vi "MongoDB.JSONtoQueryDoc.vi"(8 "error in (no error)":errorcluster, 11 "JSON Query String":string) -> (0 "error out":errorcluster, 3 ".NET Refnum out":refnum<k24>)   [LabVIEW 2014]
uses:
  C:/Users/Richard/Documents/GitHub/mongo-labview-driver/CSharp/bin/MongoDB.Driver.Legacy.dll
  CSharp/bin/MongoDB.Driver.Legacy.dll
  C:/Users/Richard/Documents/GitHub/mongo-labview-driver/CSharp/bin/MongoDB.Bson.dll
  CSharp/bin/MongoDB.Bson.dll
panel:
  out "error out 2":errorcluster
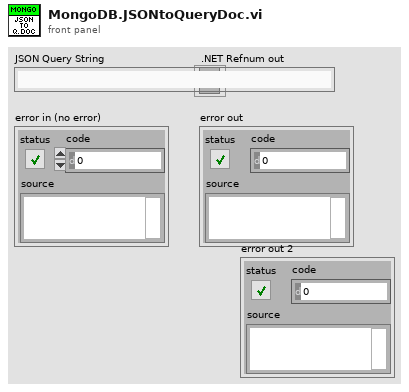
[diagram p1: front panel]
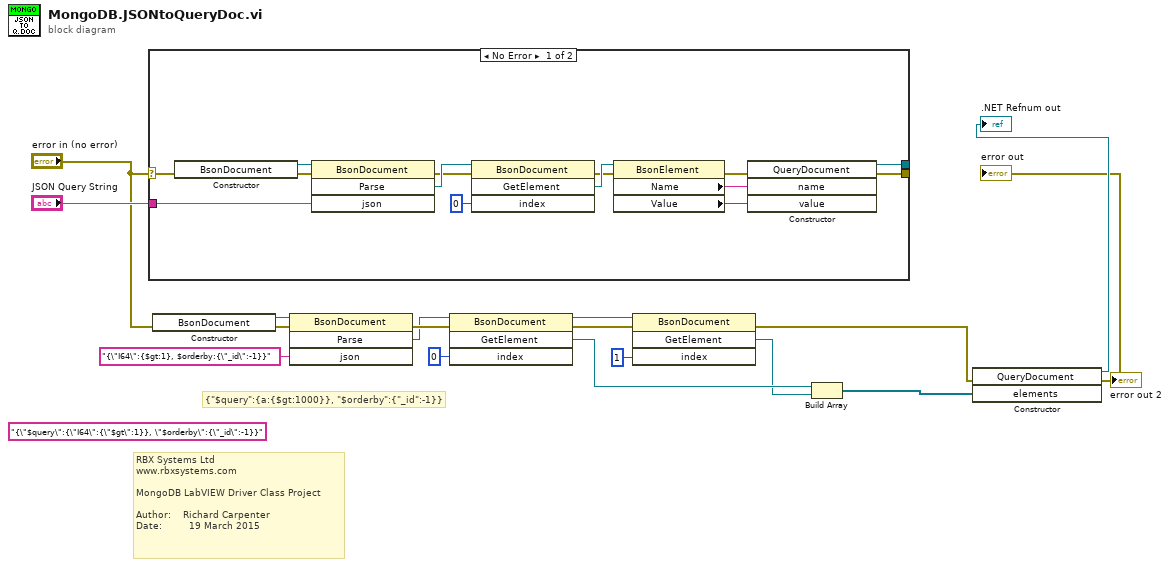
[diagram p0: block diagram]
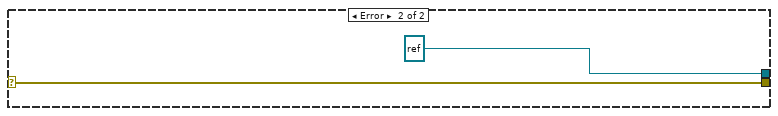
[diagram p2: hidden frame]
diagram:
  (unwired) "{\"$query\":{\"I64\":{\"$gt\":1}}, \"$orderby\":{\"_id\":-1}}" ("json")
  # "{\"$query\":{a:{$gt:1000}}, \"$orderby\":{\"_id\":-1}}"
  # "RBX Systems Ltd\nwww.rbxsystems.com\n\nMongoDB LabVIEW Driver Class Project\n\nAuthor:    Richard Carpenter\nDate:         19 March 2015"
  n1 = case shown="No Error" "error in (no error)" {
    selector: "error in (no error)" -> [w18 w33]
    tunnel: [w31 w33] -> _
    tunnel: [w30 refnum<k24> refnum ("new reference")] -> _
    tunnel: "JSON Query String" -> [w29 _]
    frame No Error {
      n2 = constructor class="BsonDocument"(error in=w18) -> (reference out=w20:refnum<k24>, error out=w19:errorcluster)  [unwired: 2 in, 1 out]
      n3 = invoke class="BsonDocument" method="Parse"(reference=w20, error in=w19, "json"=w29) -> (error out=w21:errorcluster, "Parse"=w28:refnum<k24>)  [unwired: 1 in, 2 out]
      n4 = invoke class="BsonDocument" method="GetElement"(reference=w28, error in=w21, "index"=0) -> (error out=w22:errorcluster, "GetElement"=w27:refnum<k24>)  [unwired: 1 in, 2 out]
      n5 = property class="BsonElement"(reference=w27, error in=w22) -> (error out=w23:errorcluster, "Name"=w25:string, "Value"=w26:refnum<k24>)  [unwired: 1 out]
      n6 = constructor class="QueryDocument"(error in=w23, "name"=w25, "value"=w26) -> (reference out=w30:refnum<k24>, error out=w31:errorcluster)  [unwired: 2 in, 3 out]
    }
    frame Error {
    }
  }
  n7 = constructor class="BsonDocument"(error in="error in (no error)") -> (reference out=w15:refnum<k24>, error out=w16:errorcluster)  [unwired: 2 in, 1 out]
  n8 = invoke class="BsonDocument" method="Parse"(reference=w15, error in=w16, "json"="{\"I64\":{$gt:1}, $orderby:{\"_id\":-1}}") -> (error out=w14:errorcluster, "Parse"=w10:refnum<k24>)  [unwired: 1 in, 2 out]
  n9 = invoke class="BsonDocument" method="GetElement"(reference=w10, error in=w14, "index"=0) -> (reference out=w7:refnum<k24>, error out=w3:errorcluster, "GetElement"=w11:refnum<k24>)  [unwired: 1 in, 1 out]
  n10 = invoke class="BsonDocument" method="GetElement"(reference=w7, error in=w3, "index"=1) -> (error out=w4:errorcluster, "GetElement"=w6:refnum<k24>)  [unwired: 1 in, 2 out]
  n11 = Build Array(w11, w6) -> (w9:refnum<k24>[])
  n12 = constructor class="QueryDocument"(error in=w4, "elements"=w9) -> (reference out=→".NET Refnum out":refnum<k24>, error out=→"error out" →"error out 2":errorcluster)  [unwired: 2 in, 2 out]
